vi "Test.vi"() -> ()   [LabVIEW 2018]
uses:
  Templates/Actor/Actor.lvclass
  <vilib>/Utility/error.llb/Clear Errors.vi
panel:
  out "Timeout":bool
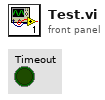
[diagram p1: front panel]
types:
  T1 = cluster{"Actor Did Initialize":refnum<event-registration>, "Actor Stopped":refnum<event-registration>}
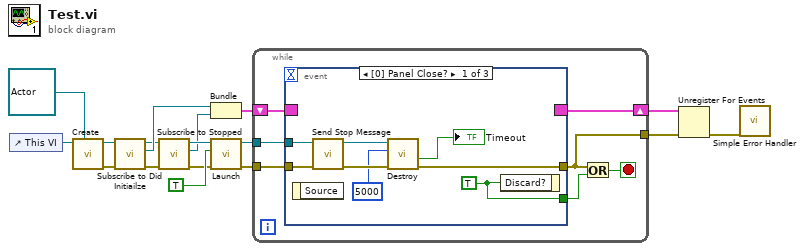
[diagram p0: block diagram]
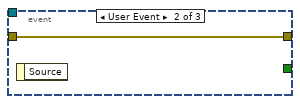
[diagram p2: hidden frame]
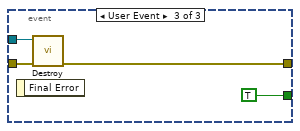
[diagram p3: hidden frame]
diagram:
  n1 = control-ref of="This VI"() -> (w4:refnum<vi>)
  n2 = call "Create.vi"("Actor in"=refnum<class "Actor.lvclass"> refnum, "Caller"=w4) -> ("error out"=w12:errorcluster, "API-Reference"=w13:refnum<data-value>)  [unwired: 8 in]
  n3 = call "Subscribe to Did Initiailze.vi"("error in (no error)"=w12, "API-Reference in"=w13) -> ("error out"=w8:errorcluster, "Actor Did Initialize"=w11:refnum<event-registration>, "API-Reference out"=w10:refnum<data-value>)  [unwired: 7 in]
  n4 = call "Subscribe to Stopped.vi"("error in (no error)"=w8, "API-Reference in"=w10) -> ("error out"=w7:errorcluster, "Actor Stopped"=w6:refnum<event-registration>, "API-Reference out"=w9:refnum<data-value>)  [unwired: 7 in]
  n5 = Bundle("Actor Did Initialize"=w11, "Actor Stopped"=w6) -> (w5:T1)  [unwired: 1 in]
  n6 = call "Launch.vi"("error in (no error)"=w7, "Show Front Panel? (F)"=TRUE, "API-Reference in"=w9) -> ("error out"=w14:errorcluster, "API-Reference out"=w15:refnum<data-value>)  [unwired: 6 in, 1 out]
  n7 = while {
    tunnel: w15 -> [w23]
    tunnel: w14 -> [w22]
    shift-right: [w24] -> w16
    shift-left: w5 -> [w21]
    tunnel: [w18] -> w2
    stop <- w19 stop-if-true
    n8 = event shown="[0] Panel Close?" {
      selector: w21 -> [_ _ _]
      dyn-events: [_ _ _] -> w24
      timeout: _ -> [_ _ _]
      tunnel: w23 -> [w31 _ w36]
      tunnel: w22 -> [w32 w33 w35]
      tunnel: [w28 w33 w34] -> w18
      tunnel: [w27 _ TRUE] -> w20
      event Panel Close? {
        w27 = TRUE
        n9 = event-data() -> ()  [unwired: 1 in, 1 out]
        n10 = call "Send Stop Message.vi"("error in (no error)"=w32, "API-Reference in"=w31) -> ("error out"=w29:errorcluster, "API-Reference out"=w30:refnum<data-value>)  [unwired: 8 in]
        n11 = call "Destroy.vi"("error in (no error)"=w29, "Wait for Stop Timeout ms (-1)"=5000, "API-Reference in"=w30) -> ("error out"=w28:errorcluster, "Timeout"=→"Timeout":bool)  [unwired: 6 in, 1 out]
        n12 = event-data("Discard?"=w27) -> ()  [unwired: 1 in, 1 out]
      }
      event User Event {
        n13 = event-data() -> ()  [unwired: 1 in, 1 out]
      }
      event User Event {
        n14 = event-data() -> ()  [unwired: 1 in, 1 out]
        n15 = call "Destroy.vi"("error in (no error)"=w35, "API-Reference in"=w36) -> ("error out"=w34:errorcluster)  [unwired: 7 in, 2 out]
      }
    }
    n16 = Or(x=w18, y=w20) -> (x .or. y?=w19:bool)
  }
  n17 = Unregister For Events(event registration refnum=w16, error in=w2) -> (error out=w1:errorcluster)
  n18 = call <vilib>:"Simple Error Handler.vi"("error in (no error)"=w1) -> ()  [unwired: 4 in, 5 out]
